vi "Ex1_Add_NET.vi"() -> ()   [LabVIEW 2013]
uses:
  D:/MATLAB_Work/NET/Ex1_add/for_testing/Ex1_add.dll
  Ex1_add/for_testing/Ex1_add.dll
panel:
  out "Sum":dbl
  in  "b":dbl
  in  "a":dbl
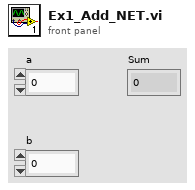
[diagram p1: front panel]
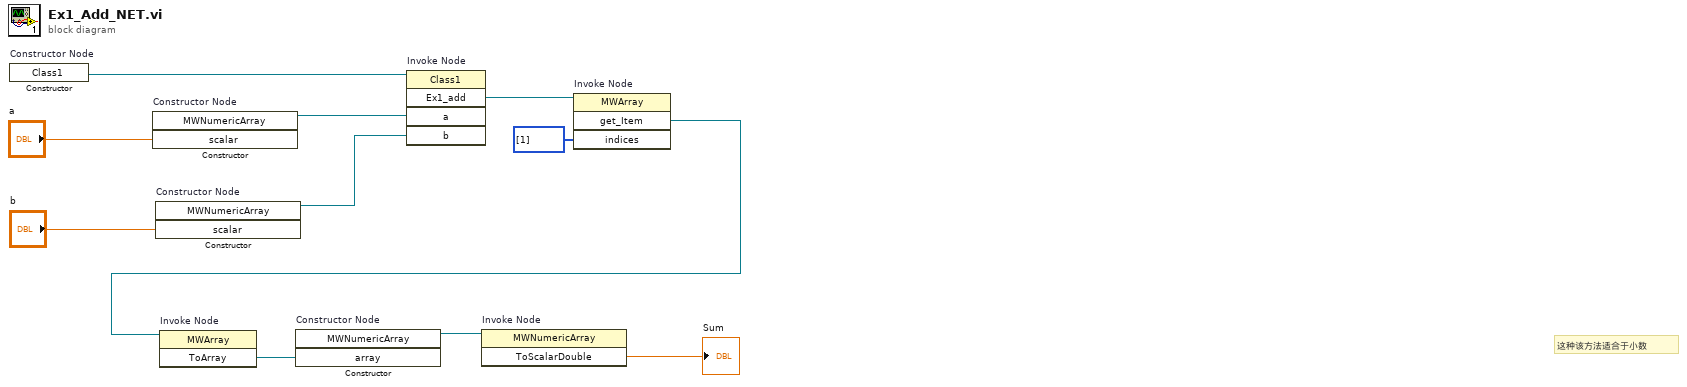
[diagram p0: block diagram]
diagram:
  # "这种该方法适合于小数"
  n1 = constructor on="Constructor Node" class="Class1"() -> (reference out=w11:refnum<k24>)  [unwired: 3 in, 2 out]
  n2 = constructor on="Constructor Node" class="MWNumericArray"("scalar"="a") -> (reference out=w10:refnum<k24>)  [unwired: 3 in, 3 out]
  n3 = constructor on="Constructor Node" class="MWNumericArray"("scalar"="b") -> (reference out=w9:refnum<k24>)  [unwired: 3 in, 3 out]
  n4 = invoke on="Invoke Node" class="Class1" method="Ex1_add"(reference=w11, "a"=w10, "b"=w9) -> ("Ex1_add"=w4:refnum<k24>)  [unwired: 2 in, 4 out]
  n5 = invoke on="Invoke Node" class="MWArray" method="get_Item"(reference=w4, "indices"=i32[] [1]) -> ("get_Item"=w1:refnum<k24>)  [unwired: 2 in, 3 out]
  n6 = invoke on="Invoke Node" class="MWArray" method="ToArray"(reference=w1) -> ("ToArray"=w5:refnum<k24>)  [unwired: 2 in, 2 out]
  n7 = constructor on="Constructor Node" class="MWNumericArray"("array"=w5) -> (reference out=w6:refnum<k24>)  [unwired: 3 in, 3 out]
  n8 = invoke on="Invoke Node" class="MWNumericArray" method="ToScalarDouble"(reference=w6) -> ("ToScalarDouble"=→"Sum":dbl)  [unwired: 2 in, 2 out]
